vi "uTTA_CreateCAL_File.vi"(4 "error in":errorcluster, 5 "Ext. called":bool, 6 "Ext. File Path":path) -> (0 "error out":errorcluster)   [LabVIEW 2021]
uses:
  <vilib>/Utility/miscctls.llb/LVPointTypeDef.ctl
  <vilib>/Utility/TDMS File Viewer/NI_TDMS File Viewer.lvlib
panel:
  out "CAL File path":path caption="selected path"
  in  "Show ADC-Cal":bool
  in  "Read uTTA-Cal":bool
  in  "Junction Calibration":T1(array[cluster]) {"Quad. Gain" format="%#_6e"; "Lin. Gain" format="%#_5e"; "Offset" format="%#_5e"}
  in  "ADC":cluster{"Offset":dbl[], "Gain":dbl[]}
  in  "PGA":cluster{"Offset":dbl[], "Gain":dbl[]}
  in  "Read ADC-Cal":bool
  in  "Write uTTA-Cal":bool
  in  "Exit":bool
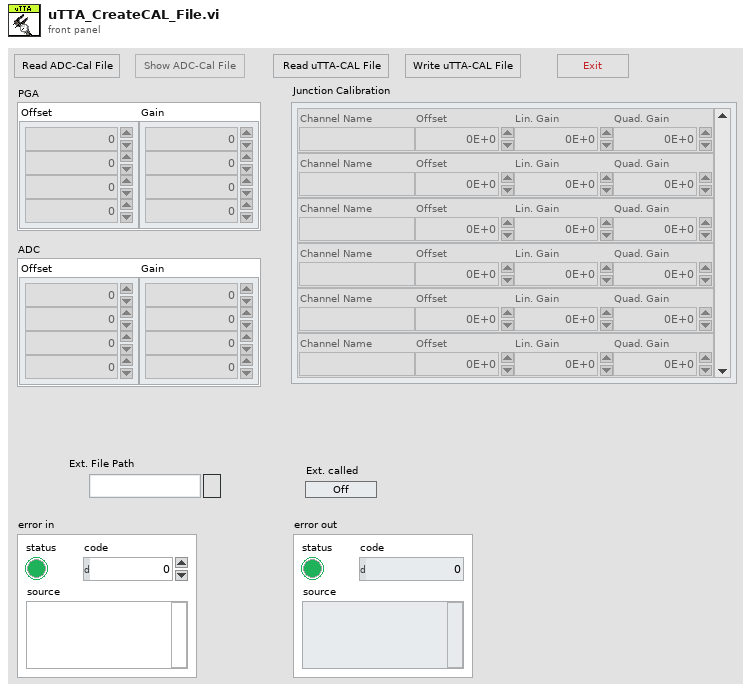
[diagram p1: front panel]
types:
  T1 = cluster{"Channel Name":string, "Offset":dbl, "Lin. Gain":dbl, "Quad. Gain":dbl}[]
  T2 = typedef "LVPointTypeDef.ctl" = cluster{"Horizontal":i16, "Vertical":i16}
  T3 = enum8{"Enabled", "Disabled", "Disabled and Grayed Out"}
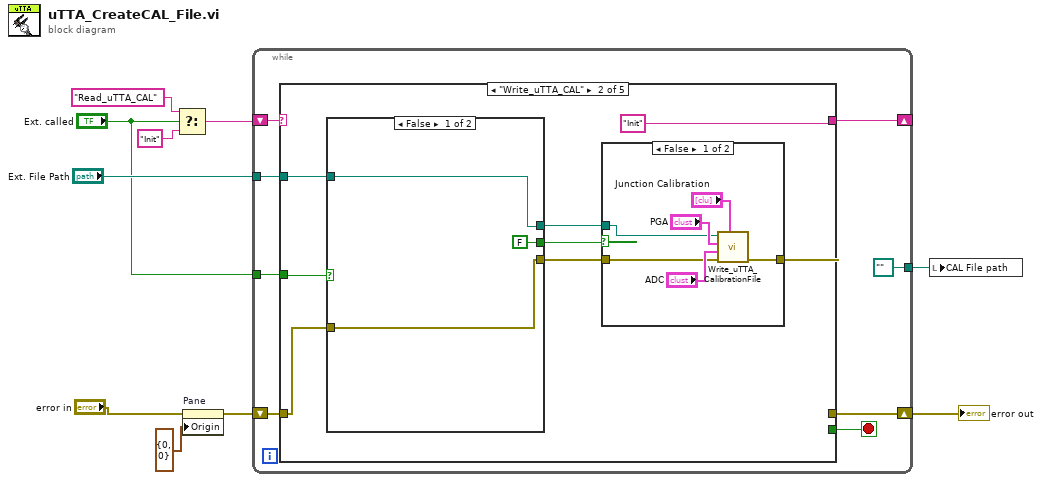
[diagram p0: block diagram]
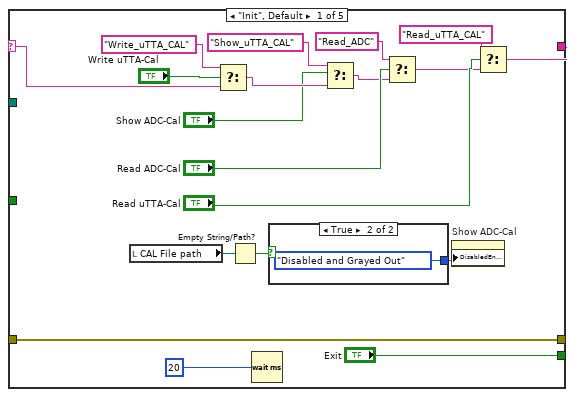
[diagram p2: hidden frame]
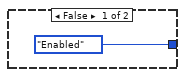
[diagram p3: hidden frame]
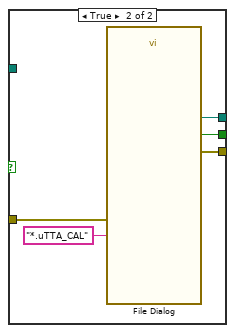
[diagram p4: hidden frame]
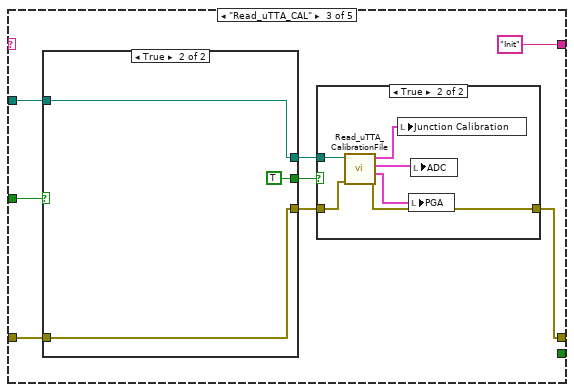
[diagram p6: hidden frame]
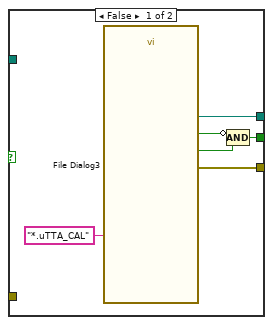
[diagram p7: hidden frame]
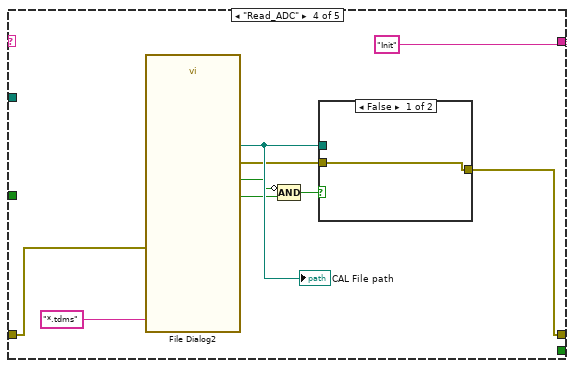
[diagram p9: hidden frame]
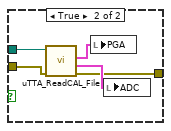
[diagram p10: hidden frame]
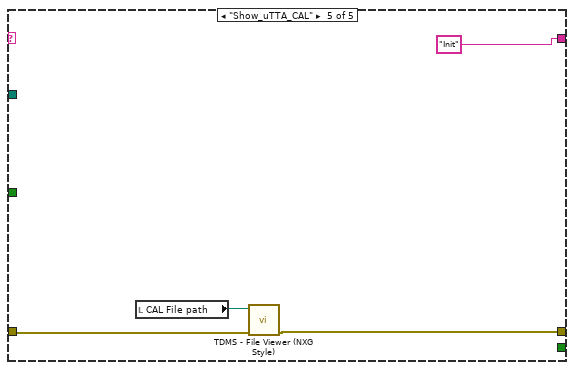
[diagram p11: hidden frame]
diagram:
  n1 = Select(t="Read_uTTA_CAL", s="Ext. called", f="Init" ("pattern (all files)")) -> (s? t:f=w4:string)
  n2 = property on="Pane" class="Pane"(error in="error in", "Origin"=T2 {"Horizontal"=0, "Vertical"=0}) -> (error out=w10:errorcluster)  [unwired: 1 in, 1 out]
  n3 = while {
    shift-right: [w17] -> _
    shift-left: w4 -> [w18]
    tunnel: [path "" ("CAL File path")] -> w8
    shift-right: [w13] -> w6
    shift-left: w10 -> [w14]
    tunnel: "Ext. File Path" -> [w12]
    tunnel: "Ext. called" -> [w11]
    stop <- w16 stop-if-true
    n4 = case shown="\"Write_uTTA_CAL\"" w18 {
      selector: w18 -> [w35 _ _ _ _]
      tunnel: [w28 "Init" ("pattern (all files)") "Init" ("pattern (all files)") "Init" ("pattern (all files)") "Init" ("pattern (all files)")] -> w17
      tunnel: ["Exit" _ _ _ _] -> w16
      tunnel: w14 -> [w19 w43 w65 w88 w103]
      tunnel: [w19 w42 w64 w87 w102] -> w13
      tunnel: w12 -> [_ w40 w63 _ _]
      tunnel: w11 -> [_ w41 w66 _ _]
      frame "Init", Default {
        n5 = local read "CAL File path"() -> (w22:path)
        n6 = Select(t="Write_uTTA_CAL", s="Write uTTA-Cal", f=w35) -> (s? t:f=w25:string)
        n7 = Empty String/Path?(string/path=w22) -> (empty?=w21:bool)
        n8 = Wait (ms)(milliseconds to wait=u32 20) -> ()  [unwired: 1 out]
        n9 = case shown="True" w21 {
          tunnel: [T3."Enabled" ("Disabled") T3."Disabled and Grayed Out" ("Disabled")] -> w20
          frame False {
          }
          frame True {
          }
        }
        n10 = Select(t="Show_uTTA_CAL", s="Show ADC-Cal", f=w25) -> (s? t:f=w24:string)
        n11 = Select(t="Read_ADC", s="Read ADC-Cal", f=w24) -> (s? t:f=w29:string)
        n12 = property on="Show ADC-Cal" class="Bool"("DisabledEnum"=w20) -> ()  [unwired: 2 in, 2 out]
        n13 = Select(t="Read_uTTA_CAL", s="Read uTTA-Cal", f=w29) -> (s? t:f=w28:string)
      }
      frame "Write_uTTA_CAL" {
        n14 = case shown="False" w41 {
          tunnel: [FALSE ("cancelled") w55] -> w47
          tunnel: [w50 w54] -> w46
          tunnel: [w48 w53] -> w45
          tunnel: w43 -> [w50 w51]
          tunnel: w40 -> [w48 _]
          frame False {
          }
          frame True {
            n15 = call "File Dialog"("error in"=w51, "pattern (all files)"="*.uTTA_CAL") -> ("selected path"=w53:path, "cancelled"=w55:bool, "error out"=w54:errorcluster)  [unwired: 10 in, 1 out]
          }
        }
        n16 = case shown="False" w47 {
          tunnel: w46 -> [w58 w62]
          tunnel: w45 -> [w59 _]
          tunnel: [w56 w62] -> w42
          frame False {
            n17 = call "Write_uTTA_CalibrationFile.vi"("Junction Calibration"="Junction Calibration", "error in (no error)"=w58, "ADC"="ADC", "PGA"="PGA", "selected path"=w59) -> ("error out"=w56:errorcluster)  [unwired: 6 in]
          }
          frame True {
          }
        }
      }
      frame "Read_uTTA_CAL" {
        n18 = case shown="True" w66 {
          tunnel: [w76 w78] -> w70
          tunnel: [w75 w77] -> w69
          tunnel: [w71 TRUE] -> w67
          tunnel: w65 -> [_ w78]
          tunnel: w63 -> [_ w77]
          frame False {
            n19 = call "File Dialog3"("pattern (all files)"="*.uTTA_CAL") -> ("selected path"=w75:path, "exists"=w73:bool, "cancelled"=w72:bool, "error out"=w76:errorcluster)  [unwired: 11 in]
            n20 = Compound Arithmetic op=AND(invert w72, w73) -> (w71:bool)
          }
          frame True {
          }
        }
        n21 = case shown="True" w67 {
          tunnel: w70 -> [w80 w85]
          tunnel: w69 -> [_ w86]
          tunnel: [w80 w81] -> w64
          frame False {
          }
          frame True {
            n22 = call "Read_uTTA_CalibrationFile.vi"("error in (no error)"=w85, "selected path"=w86) -> ("error out"=w81:errorcluster, "PGA"=w83:cluster{"Offset":dbl[], "Gain":dbl[]}, "ADC"=w82:cluster{"Offset":dbl[], "Gain":dbl[]}, "Channels"=w84:T1)  [unwired: 6 in]
            n23 = local write "Junction Calibration"(w84) -> ()
            n24 = local write "PGA"(w83) -> ()
            n25 = local write "ADC"(w82) -> ()
          }
        }
      }
      frame "Read_ADC" {
        n26 = call "File Dialog2"("error in"=w88, "pattern (all files)"="*.tdms") -> ("selected path"=w93:path, "exists"=w92:bool, "cancelled"=w91:bool, "error out"=w89:errorcluster)  [unwired: 10 in]
        "CAL File path" <- w93
        n27 = Compound Arithmetic op=AND(invert w91, w92) -> (w90:bool)
        n28 = case shown="False" w90 {
          tunnel: w93 -> [_ w101]
          tunnel: w89 -> [w96 w100]
          tunnel: [w96 w97] -> w87
          frame False {
          }
          frame True {
            n29 = call "uTTA_ReadCAL_File.vi"("error in"=w100, "file path"=w101) -> ("error out"=w97:errorcluster, "ADC"=w98:cluster{"Offset":dbl[], "Gain":dbl[]}, "PGA"=w99:cluster{"Offset":dbl[], "Gain":dbl[]})  [unwired: 7 in]
            n30 = local write "PGA"(w99) -> ()
            n31 = local write "ADC"(w98) -> ()
          }
        }
      }
      frame "Show_uTTA_CAL" {
        n32 = local read "CAL File path"() -> (w104:path)
        n33 = call <vilib>:"TDMS - File Viewer (NXG Style).vi"("error in"=w103, "file in"=w104) -> ("error out"=w102:errorcluster)  [unwired: 8 in, 1 out]
      }
    }
  }
  "error out" <- w6
  n34 = local write "CAL File path"(w8) -> ()
